vi "log_error.vi"(6 "timestamp":timestamp, 7 "context":string, 8 "error in (no error)":errorcluster, 9 "level":T1=200 items=["OFF"=0, "FATAL"=100, "ERROR"=200, "WARN"=300, "INFO"=400, "DEBUG"=500, "TRACE"=600, "ALL"=65535], 11 "Queue Log Provider in":refnum<class "Queue Log Provider.lvclass">) -> (0 "error out":errorcluster, 3 "Queue Log Provider out":refnum<class "Queue Log Provider.lvclass">)   [LabVIEW 2019, in "LVCOOOP.lvlib" / "Support API.lvlib" / "Queue Log Provider.lvclass"]
uses:
  Queue Log Provider.lvclass
  Log Service/public/level.ctl
  log_message.ctl
  Queue Log Provider.lvclass/Queue Log Provider.ctl
  Log Service/Log Service.lvclass
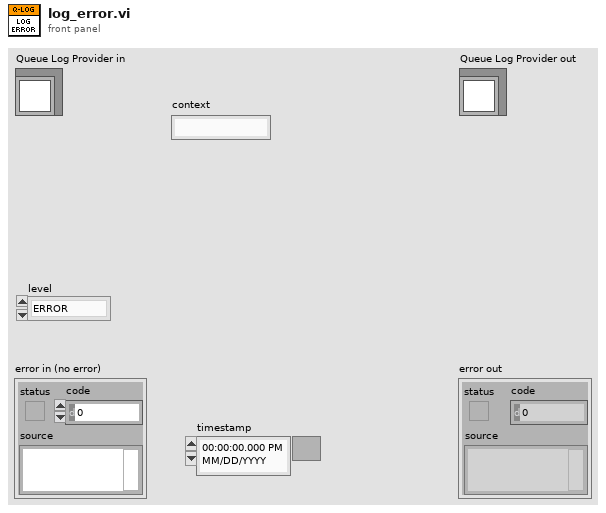
[diagram p1: front panel]
types:
  T1 = typedef "LVCOOOP.lvlib/Support API.lvlib/Log Service.lvclass/level.ctl" = u16
  T2 = typedef "LVCOOOP.lvlib/Support API.lvlib/Queue Log Provider.lvclass/log_message.ctl" = cluster{"Time Stamp":timestamp, "level":T1, "context":string, "message":string}
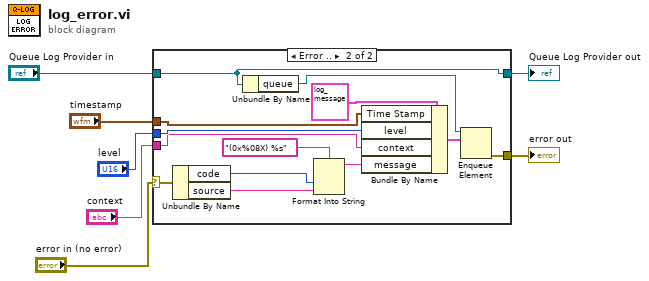
[diagram p0: block diagram]
diagram:
  n1 = case shown="Error .." "error in (no error)" {
    selector: "error in (no error)" -> [w9 w14]
    tunnel: [w9 w21] -> w1
    tunnel: "timestamp" -> [_ w19]
    tunnel: "level" -> [_ w18]
    tunnel: "context" -> [_ w17]
    tunnel: [w8 w15] -> w5
    tunnel: "Queue Log Provider in" -> [w8 w15]
    frame No Error {
    }
    frame Error {
      n2 = Unbundle By Name(w14) -> ("code"=w12:i32, "source"=w11:string)
      n3 = Unbundle By Name(w15) -> ("queue"=w22:refnum<queue>)
      n4 = Format Into String(format string="(0x%08X) %s", w12, w11) -> (resulting string=w10:string)  [unwired: 2 in, 1 out]
      n5 = Bundle By Name(cluster=T2 {"Time Stamp"=timestamp(0 s since 1904-01-01), "level"=0, "context"="", "message"=""} ("element"), "Time Stamp"=w19, "level"=w18, "context"=w17, "message"=w10) -> (w16:T2)
      n6 = Enqueue Element(queue=w22, element=w16) -> (error out=w21:errorcluster)  [unwired: 2 in, 2 out]
    }
  }
  "error out" <- w1
  "Queue Log Provider out" <- w5
